vi "CheckWavenameLength.vi"(1 "wavename":string) -> (0 "wavename":string)   [LabVIEW 2016, in "LVtoITX.lvclass"]
uses:
  LVtoITX.lvclass
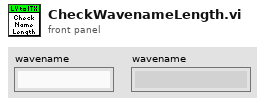
[diagram p1: front panel]
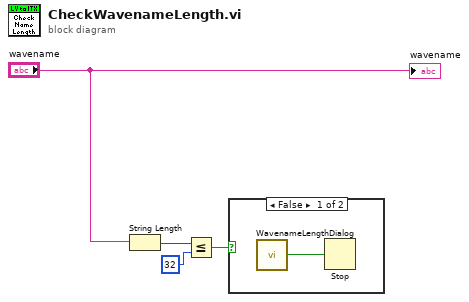
[diagram p0: block diagram]
diagram:
  n1 = String Length(string="wavename") -> (length=w2:i32)
  n2 = Less Or Equal?(x=w2, y=32) -> (x <= y?=w4:bool)
  n3 = case shown="False" w4 {
    frame False {
      n4 = call "WavenameLengthDialog.vi"() -> ("Boolean 2"=w5:bool)
      n5 = Stop(stop? (T)=w5) -> ()
    }
    frame True {
    }
  }
  "wavename" <- "wavename"
